vi "motor_done_moving.vi"(10 "wait at least (s)":dbl=2.0) -> ()   [LabVIEW 2013]
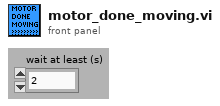
[diagram p1: front panel]
types:
  T1 = enum16{"GET STATUS", "ABS MOVE", "GET POS", "REL MOVE", "INIT", "CLOSE", "HOME", "READ ASCII", "ASCII", "SET ULIM", "STOP", "SET LLIM"}
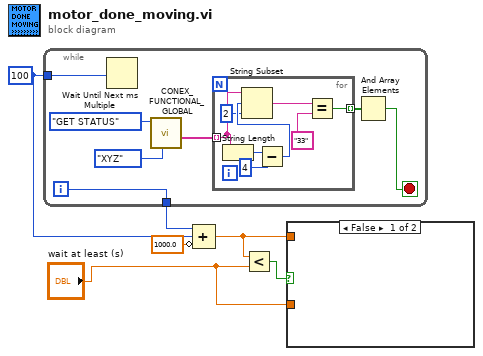
[diagram p0: block diagram]
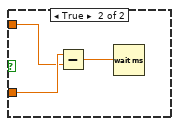
[diagram p2: hidden frame]
diagram:
  w5 = u32 100 ("milliseconds to wait")
  n1 = while {
    tunnel: [w8] -> w6
    tunnel: w5 -> [w7]
    i -> [w8]
    stop <- w10 stop-if-true
    n2 = Wait Until Next ms Multiple(millisecond multiple=w7) -> ()  [unwired: 1 out]
    n3 = call "CONEX_FUNCTIONAL_GLOBAL.vi"("Axis"=enum16{"X", "Y", "Z", "XY", "XZ", "YZ", "XYZ"}."XYZ", "Command"=T1."GET STATUS") -> ("ASCII response"=w12:string[])  [unwired: 7 in, 2 out]
    n4 = for {
      tunnel: w12 -> [w21] mode=indexing
      tunnel: [w15] -> w11 mode=indexing
      n5 = String Length(string=w21) -> (length=w20:i32)
      n6 = Subtract(x=w20, y=4) -> (x-y=w18:i32)
      n7 = String Subset(string=w21, offset (0)=w18, length (rest)=2 ("length (rest)")) -> (substring=w17:string)
      n8 = Equal?(x=w17, y="33") -> (x = y?=w15:bool)
    }
    n9 = And Array Elements(Boolean array=w11) -> (logical AND=w10:bool)
  }
  n10 = Compound Arithmetic op=unknown(w6, w5, invert 1000.0 ("value")) -> (w1:dbl)
  n11 = Less?(x=w1, y="wait at least (s)") -> (x < y?=w3:bool)
  n12 = case shown="False" w3 {
    tunnel: "wait at least (s)" -> [_ w24]
    tunnel: w1 -> [_ w23]
    frame False {
    }
    frame True {
      n13 = Subtract(x=w24, y=w23) -> (x-y=w22:dbl)
      n14 = Wait (ms)(milliseconds to wait=w22) -> ()  [unwired: 1 out]
    }
  }
